vi "Clear Read Buffer.vi"(8 "error in (no error)":errorcluster, 11 "RP Communicator in":refnum<class "RP Communicator.lvclass">) -> (0 "error out":errorcluster, 1 "bytes read":i32, 2 "data out":string, 3 "RP Communicator out":refnum<class "RP Communicator.lvclass">, 4 "hex bytes":string, 5 "Call log":string, 6 "Server address":string="192.168.1.100")   [LabVIEW 2024, in "RP Communicator.lvclass"]
uses:
  RP Communicator.lvclass
  RP Communicator.lvclass/RP Communicator.ctl
  Controls/RP Com Log.ctl
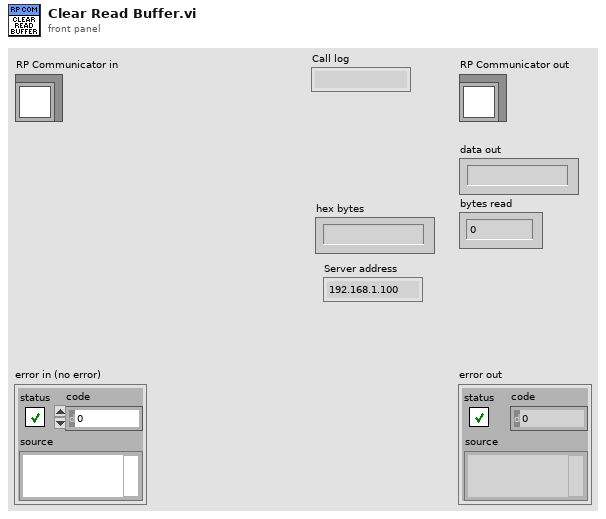
[diagram p1: front panel]
types:
  T1 = typedef "RP Com Log.ctl" = cluster{"in length":i32, "out length":i32, "in value":u64, "out  value":u64}
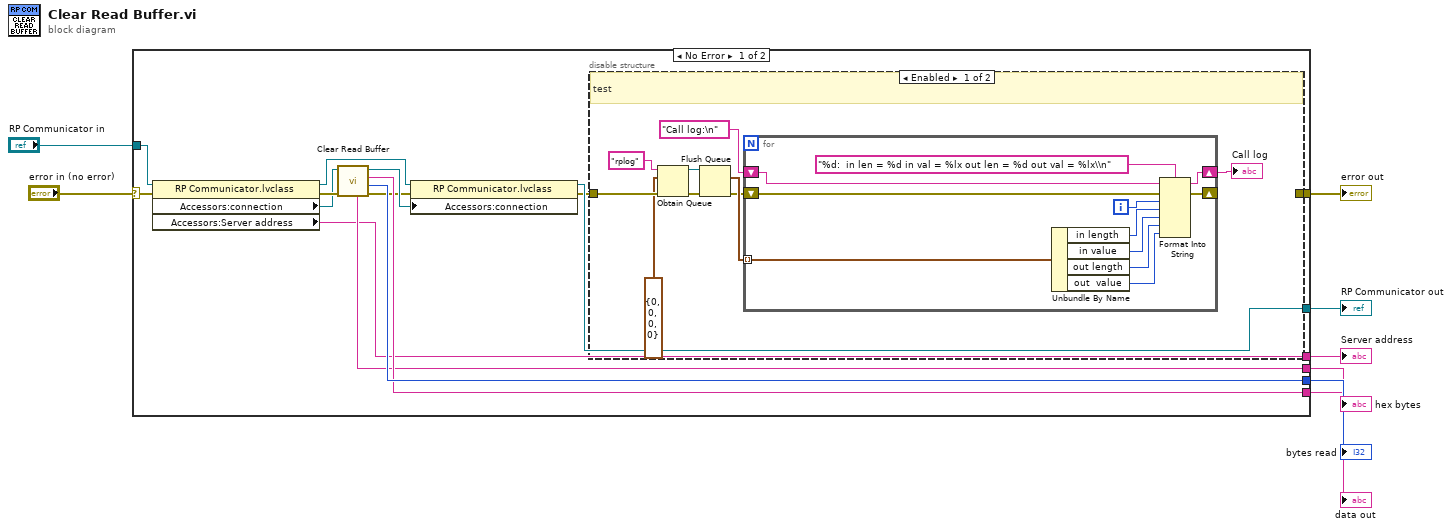
[diagram p0: block diagram]
diagram:
  n1 = case shown="No Error" "error in (no error)" {
    selector: "error in (no error)" -> [w18 w45]
    tunnel: [w9 w45] -> w7
    tunnel: [w20 w44] -> w5
    tunnel: "RP Communicator in" -> [w22 w44]
    tunnel: [w15 _] -> w4
    tunnel: [w14 _] -> w3
    tunnel: [w13 _] -> w2
    tunnel: [w12 _] -> w1
    frame No Error {
      n2 = property class="RP Communicator.lvclass"(reference=w22, error in=w18) -> (reference out=w21:refnum<class "RP Communicator.lvclass">, error out=w19:errorcluster, "Accessors:connection"=w17:refnum<k5>, "Accessors:Server address"=w12:string)
      n3 = call "Clear Read Buffer.vi"("error in"=w19, "connection ID"=w17) -> ("error out"=w11:errorcluster, "bytes read"=w15:i32, "data out"=w14:string, "connection ID out"=w16:refnum<k5>, "hex bytes"=w13:string)  [unwired: 5 in]
      n4 = property class="RP Communicator.lvclass"(reference=w21, error in=w11, "Accessors:connection"=w16) -> (reference out=w20:refnum<class "RP Communicator.lvclass">, error out=w10:errorcluster)
      n5 = disable-structure shown="Enabled" {
        disable-tunnel: w10 -> [w28 w43]
        disable-tunnel: [_ w43] -> w9
        frame Enabled {
          # "test"
          n6 = Obtain Queue(name (unnamed)="rplog", element data type=T1 {"in length"=0, "out length"=0, "in value"=0, "out  value"=0} ("RP com log"), error in (no error)=w28) -> (queue out=w29:refnum<queue>, error out=w30:errorcluster)  [unwired: 2 in, 1 out]
          n7 = Flush Queue(queue=w29, error in (no error)=w30) -> (remaining elements=w27:T1[], error out=w26:errorcluster)  [unwired: 1 out]
          n8 = for {
            tunnel: w27 -> [w42] mode=indexing
            shift-right: [w41] -> _
            shift-left: w26 -> [w40]
            shift-right: [w37] -> w23
            shift-left: "Call log:\n" ("format string") -> [w38]
            i -> [w36]
            n9 = Unbundle By Name(w42) -> ("in length"=w35:i32, "in value"=w34:u64, "out length"=w33:i32, "out  value"=w32:u64)
            n10 = Format Into String(format string="%d:  in len = %d in val = %lx out len = %d out val = %lx\\n", initial string=w38, error in=w40, w36, w35, w34, w33, w32) -> (resulting string=w37:string, error out=w41:errorcluster)
          }
          "Call log" <- w23
        }
        frame Disabled {
          # "run"
        }
      }
    }
    frame Error {
    }
  }
  "error out" <- w7
  "RP Communicator out" <- w5
  "bytes read" <- w4
  "data out" <- w3
  "hex bytes" <- w2
  "Server address" <- w1
